vi "ROOT - Obtain Session.vi"(0 "Session Name ()":string, 2 "OBJ - Session":refnum<class "Session - Root.lvclass">, 11 "error in (no error)":errorcluster) -> (4 "Session Handle":T1, 8 "created new?":bool, 15 "error out":errorcluster)   [LabVIEW 2015, in "Session - Root.lvclass"]
doc: "Obtains a reference to a session.\nIf session exists, vi returns active reference.\nIf session does not exist, vi runs 'set Defaults.vi' of session class hierarchy."
uses:
  Session - Root.lvclass
  Typedefs/Session Handle.ctl
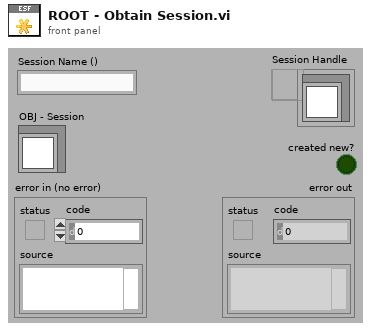
[diagram p1: front panel]
types:
  T1 = typedef "Session - Root.lvclass/Session Handle.ctl" = refnum<data-value>
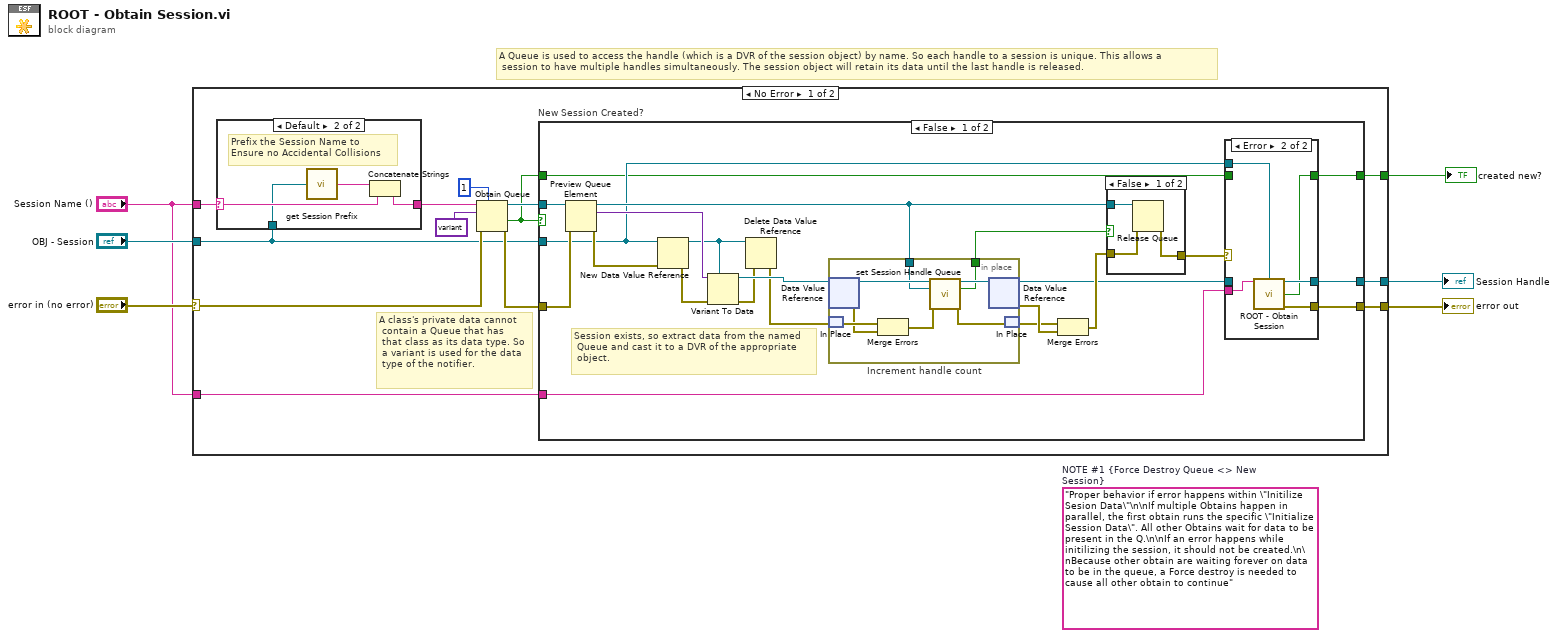
[diagram p0: block diagram]
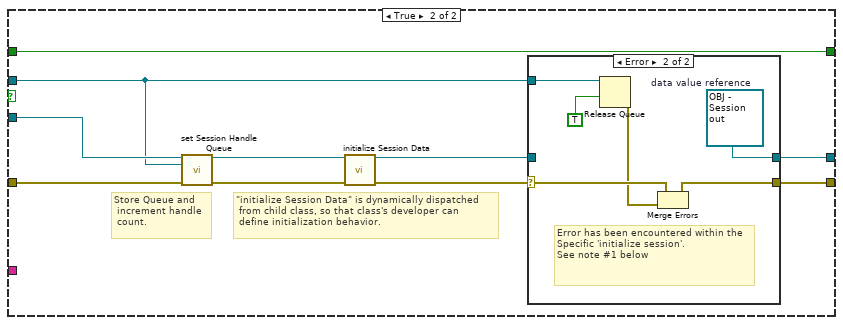
[diagram p5: hidden frame]
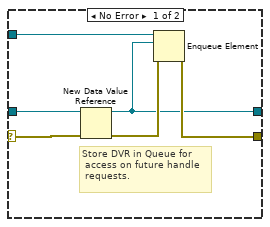
[diagram p6: hidden frame]
diagram:
  (unwired) "Proper behavior if error happens within \"Initilize Sesion Data\"\n\nIf multiple Obtains happen in parallel, the first obtain runs the specific \"Initialize Session Data\". All other Obtains wait for data to be present in the Q.\n\nIf an error happens while initilizing the session, it should not be created.\n\nBecause other obtain are waiting forever on data to be in the queue, a Force destroy is needed to cause all other obtain to continue"  # NOTE #1 {Force Destroy Queue <> New Session}
  # "A Queue is used to access the handle (which is a DVR of the session object) by name. So each handle to a session is unique. This allows a\n session to have multiple handles simultaneously. The session object will retain its data until the last handle is released."
  n1 = case shown="No Error" "error in (no error)" {
    selector: "error in (no error)" -> [w19 w89]
    tunnel: [w18 w89] -> w5
    tunnel: [w17 _] -> w4
    tunnel: "Session Name ()" -> [w13 _]
    tunnel: "OBJ - Session" -> [w14 _]
    tunnel: [w9 _] -> w2
    tunnel: "Session Name ()" -> [w7 _]
    frame No Error {
      # "A class's private data cannot\n contain a Queue that has\n that class as its data type. So\n a variant is used for the data\n type of the notifier."
      n2 = case shown="Default" w13 {
        selector: w13 -> [w20 w23]
        tunnel: [w20 w24] -> w11
        tunnel: w14 -> [_ w22]
        frame "" {
        }
        frame Default {
          # "Prefix the Session Name to Ensure no Accidental Collisions"
          n3 = call-dynamic "get Session Prefix.vi"("Session - Root"=w22) -> ("Session Prefix"=w21:string)  [unwired: 14 in]
          n4 = Concatenate Strings(w21, w23) -> (w24:string)
        }
      }
      n5 = Obtain Queue(max queue size (-1, unlimited)=1, name (unnamed)=w11, element data type=variant ("Variant"), error in (no error)=w19) -> (queue out=w16:refnum<queue>, created new?=w8:bool, error out=w15:errorcluster)  [unwired: 1 in]
      n6 = case "New Session Created?" shown="False" w8 {
        tunnel: w15 -> [w45 w75]
        tunnel: [w29 w76] -> w18
        tunnel: [w30 w71] -> w17
        tunnel: w16 -> [w46 w69]
        tunnel: w14 -> [w27 w74]
        tunnel: [w26 w67] -> w9
        tunnel: w8 -> [w25 w67]
        tunnel: w7 -> [w32 _]
        frame False {
          # "Session exists, so extract data from the named\n Queue and cast it to a DVR of the appropriate\n object."
          n7 = Preview Queue Element(queue=w46, error in (no error)=w45) -> (queue out=w43:refnum<queue>, element=w44:variant, error out=w42:errorcluster)  [unwired: 1 in, 1 out]
          n8 = New Data Value Reference(data value=w27, error in=w42) -> (data value reference=w39:refnum<data-value>, error out=w40:errorcluster)
          n9 = Variant To Data(error in=w40, type=w39, Variant=w44) -> (data=w38:refnum<data-value>, error out=w35:errorcluster)
          n10 = Delete Data Value Reference(data value reference=w39, error in=w35) -> (error out=w34:errorcluster)  [unwired: 1 out]
          n11 = in-place "Increment handle count" {
            in-place-border: w43 -> [w60]
            in-place-border: [w59] -> w36
            n12 = in-place-dvr #1(w38) -> (w66:refnum<class "Session - Root.lvclass">, w62:errorcluster)
            n13 = in-place-match #2(w34) -> (w63:errorcluster)
            n14 = Merge Errors(w63, w62) -> (w61:errorcluster)
            n15 = call "set Session Handle Queue.vi"("OBJ - Session in"=w66, "Session Queue Handle"=w60, "error in (no error)"=w61) -> ("OBJ - Session out"=w65:refnum<class "Session - Root.lvclass">, "Stored new reference"=w59:bool, "error out"=w64:errorcluster)  [unwired: 10 in]
            n16 = in-place-dvr #1(w65) -> (w28:refnum<data-value>, w41:errorcluster)
            n17 = in-place-match #2(w64) -> (w37:errorcluster)
          }
          n18 = Merge Errors(w37, w41) -> (w33:errorcluster)
          n19 = case shown="False" w36 {
            tunnel: w33 -> [w56 w58]
            tunnel: w43 -> [w57 _]
            tunnel: [w55 w58] -> w31
            frame False {
              n20 = Release Queue(queue=w57, error in (no error)=w56) -> (error out=w55:errorcluster)  [unwired: 1 in, 2 out]
            }
            frame True {
            }
          }
          n21 = case shown="Error" w31 {
            selector: w31 -> [w48 _]
            tunnel: w32 -> [_ w54]
            tunnel: [w49 w53] -> w30
            tunnel: [w48 w52] -> w29
            tunnel: w27 -> [_ w51]
            tunnel: w28 -> [w49 _]
            tunnel: [w47 w50] -> w26
            tunnel: w25 -> [w47 _]
            frame No Error {
            }
            frame Error {
              n22 = call "ROOT - Obtain Session.vi"("Session Name ()"=w54, "OBJ - Session"=w51) -> ("Session Handle"=w53:T1, "created new?"=w50:bool, "error out"=w52:errorcluster)  [unwired: 11 in]
            }
          }
        }
        frame True {
          # "Store Queue and\n increment handle\n count."
          # "\"initialize Session Data\" is dynamically dispatched\n from child class, so that class's developer can\n define initialization behavior."
          n23 = call "set Session Handle Queue.vi"("OBJ - Session in"=w74, "Session Queue Handle"=w69, "error in (no error)"=w75) -> ("OBJ - Session out"=w73:refnum<class "Session - Root.lvclass">, "error out"=w72:errorcluster)  [unwired: 10 in, 1 out]
          n24 = call-dynamic "initialize Session Data.vi"("OBJ - Session in"=w73, "error in"=w72) -> ("OBJ - Session out"=w70:refnum<class "Session - Root.lvclass">, "error out"=w68:errorcluster)  [unwired: 12 in]
          n25 = case shown="Error" w68 {
            selector: w68 -> [w77 w85]
            tunnel: [w82 w83] -> w76
            tunnel: [w80 w87] -> w71
            tunnel: w70 -> [w79 _]
            tunnel: w69 -> [w78 w88]
            frame No Error {
              # "Store DVR in Queue for\n access on future handle\n requests."
              n26 = New Data Value Reference(data value=w79, error in=w77) -> (data value reference=w80:refnum<data-value>, error out=w81:errorcluster)
              n27 = Enqueue Element(queue=w78, element=w80, error in (no error)=w81) -> (error out=w82:errorcluster)  [unwired: 1 in, 2 out]
            }
            frame Error {
              w87 = refnum<data-value> refnum  # data value reference
              # "Error has been encountered within the Specific 'initialize session'.\nSee note #1 below"
              n28 = Release Queue(queue=w88, force destroy? (F)=TRUE) -> (error out=w84:errorcluster)  [unwired: 1 in, 2 out]
              n29 = Merge Errors(w85, w84) -> (w83:errorcluster)
            }
          }
        }
      }
    }
    frame Error {
    }
  }
  "error out" <- w5
  "Session Handle" <- w4
  "created new?" <- w2
